vi "Climb.vi"(7 "Description":string, 8 "Command Info In":T3, 11 "SubSystem Data":T1) -> (0 "Command Info Out":T3)   [LabVIEW 2020]
doc: "This template is useful for immediate subsystem actions that do not need deadband filtering\n\nBe sure to right-click and select New from Template and save with a new command name."
uses:
  <vilib>/Rock Robotics/WPI/Framework/Command Status Info.ctl
  <vilib>/Rock Robotics/WPI/Framework/Completion Status.ctl
  <vilib>/Rock Robotics/WPI/Framework/Completion Notifier.ctl
  Implementation/Climber Setpoints.ctl
  Implementation/Climber Operations.ctl
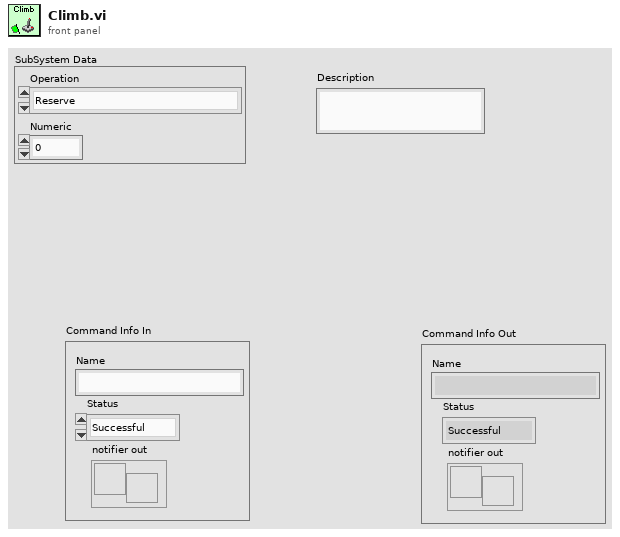
[diagram p1: front panel]
types:
  T1 = typedef "Climber Setpoints.ctl" = cluster{"Operation":T2, "Numeric":dbl}
  T2 = typedef "Climber Operations.ctl" = enum16{"Reserve", "Read Current", "Immediate", "Unlock Winch", "Lock Winch", "Stop Winch", "Spool Winch", "Unspool Winch", "Arm Out", "Arm In", "Open Hook", "Close Hook"}
  T3 = typedef "Command Status Info.ctl" = cluster{"Name":string, "Status":T4, "notifier out":T5}
  T4 = typedef "Completion Status.ctl" = enum16{"Successful", "Aborted", "Incomplete"}
  T5 = typedef "Completion Notifier.ctl" = refnum<notifier>
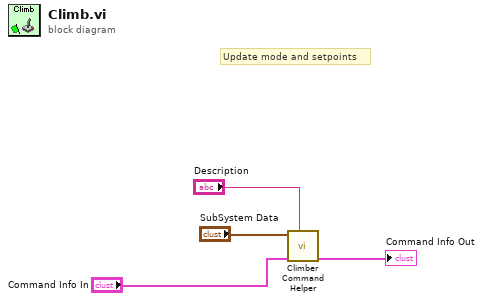
[diagram p0: block diagram]
diagram:
  # "Update mode and setpoints"
  n1 = call "Climber Command Helper.vi"("Description"="Description", "Command Info In"="Command Info In", "SubSystem Data"="SubSystem Data") -> ("Command Info Out"=→"Command Info Out":T3)  [unwired: 6 in, 2 out]
